vi "prueba camera control.vi"() -> ()   [LabVIEW 2010]
uses:
  <vilib>/addons/PixeLINK/Low Level Functions/CAMERA_FEATURES.llb/TDPU-CameraFeatures-PixelFormat.ctl
  <vilib>/vision/Image Controls.llb/IMAQ Image.ctl
panel:
  in  "Mostrar?":bool
  out "Image Device OUT":cluster{"Image":T1, "errorImage":errorcluster}
  in  "Camera Parameters":T3 {"Pixel Format" items=["PIXEL_FORMAT_MONO8", "PIXEL_FORMAT_MONO16", "PIXEL_FORMAT_YUV422", "PIXEL_FORMAT_BAYER8_GRBG", "PIXEL_FORMAT_BAYER16_GRBG", "PIXEL_FORMAT_RGB24", "PIXEL_FORMAT_RGB48", "PIXEL_FORMAT_BAYER8_RGGB", "PIXEL_FORMAT_BAYER8_GBRG ", "PIXEL_FORMAT_BAYER8_BGGR ", "PIXEL_FORMAT_BAYER16_RGGB ", "PIXEL_FORMAT_BAYER16_GBRG", "PIXEL_FORMAT_BAYER16_BGGR", "PIXEL_FORMAT_RGB32"]}
  in  "Selector":u16(ring) items=["776002034"]
  in  "stop":bool
  in  "Streeam?":bool
  out "Image":T1(plugin-control)
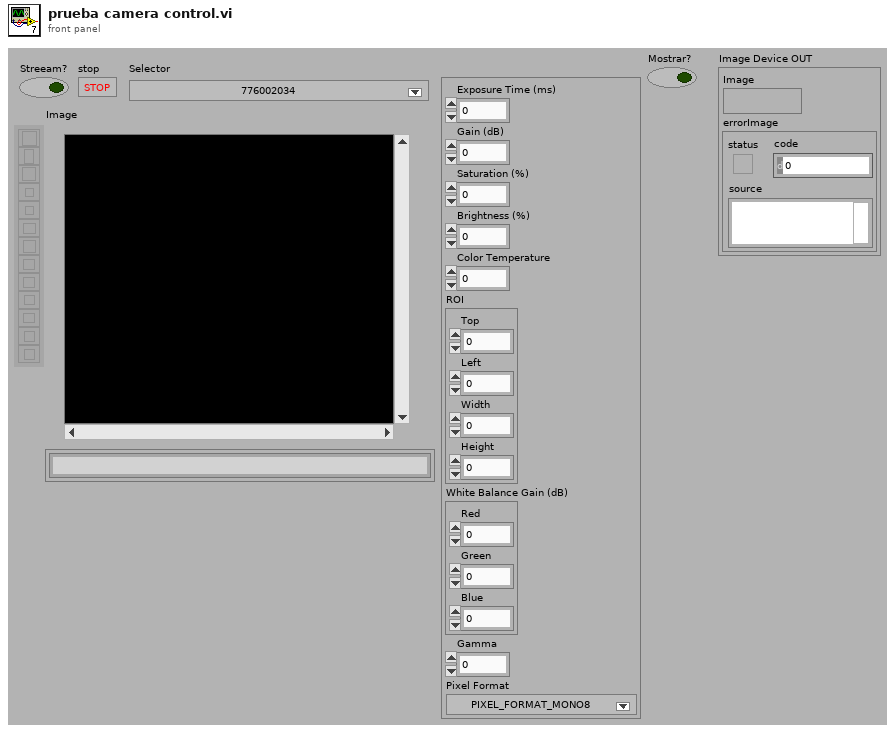
[diagram p1: front panel]
types:
  T1 = typedef "IMAQ Image.ctl" = refnum<image>
  T2 = typedef "TDPU-CameraFeatures-PixelFormat.ctl" = u16
  T3 = cluster{"Exposure Time (ms)":u32, "Gain (dB)":dbl, "Saturation (%)":dbl, "Brightness (%)":dbl, "Color Temperature":dbl, "ROI":cluster{"Top":i32, "Left":i32, "Width":i32, "Height":i32}, "White Balance Gain (dB)":cluster{"Red":dbl, "Green":dbl, "Blue":dbl}, "Gamma":dbl, "Pixel Format":T2}
  T4 = cluster{"hCamera":u32, "Error":errorcluster, "uSerialNumber OUT":u32}
  T5 = cluster{"hCamera":u32, "Error":errorcluster, "uSerialNumber":u32}
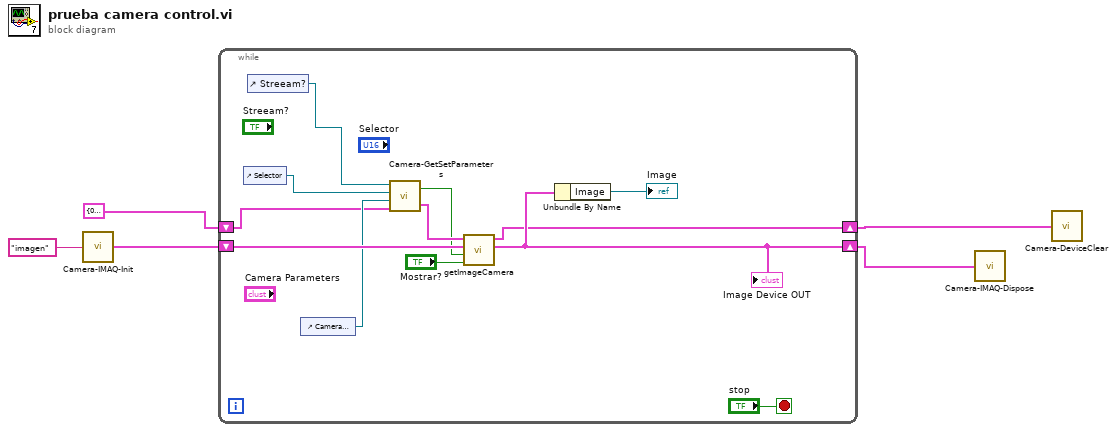
[diagram p0: block diagram]
diagram:
  n1 = call "Camera-IMAQ-Init.vi"("Image Name"="imagen") -> ("Image Device IN"=w4:cluster{"Image":T1, "errorImage":errorcluster})
  n2 = while {
    shift-right: [w12] -> w1
    shift-left: w4 -> [w15]
    shift-right: [w10] -> w2
    shift-left: T4 {"hCamera"=0, "Error"={"status"=FALSE, "code"=0, "source"=""}, "uSerialNumber OUT"=0} ("Camera Device  IN") -> [w9]
    stop <- "stop" stop-if-true
    n3 = control-ref of="Selector"() -> (w14:refnum<vi>)
    n4 = control-ref of="Streeam?"() -> (w11:refnum<vi>)
    n5 = control-ref of="Camera Parameters"() -> (w13:refnum<vi>)
    n6 = call "Camera-GetSetParameters.vi"("Camera Device  IN"=w9, "Camera Parameters"=w13, "Selector"=w14, "Stream?"=w11) -> ("Camera Device OUT"=w7:T5, "Stream? OUT"=w6:bool)
    n7 = call "getImageCamera.vi"("Mostrar?"="Mostrar?", "Streeam?"=w6, "Image Device IN"=w15, "Camera Device  IN"=w7) -> ("Image Device OUT"=w12:cluster{"Image":T1, "errorImage":errorcluster}, "Camera Device OUT"=w10:T4)  [unwired: 1 in, 1 out]
    "Image Device OUT" <- w12
    n8 = Unbundle By Name(w12) -> ("Image"=→"Image":T1)
  }
  n9 = call "Camera-IMAQ-Dispose.vi"("Image Device IN"=w1) -> ()
  n10 = call "Camera-DeviceClear.vi"("Camera Device OUT"=w2) -> ()
